vi "Yahoo - Get Data (for stock ticker).vi"(0 "Symbol":string, 3 "error in":errorcluster) -> (6 "Stock Data":T1, 9 "error out":errorcluster)   [LabVIEW 2011]
doc: "Get the symbol data from Yahoo Finance.\n\nInputs:\n Symbol: Stock ticker symbol.\n Error in: Describes error conditions that occur before this node runs. This input provides standard error in functionality.\n\nOutputs:\n Stock Data: Parsed Stock Data\n Symbol\n Name\n Price\n Change\n Change %\n Volume: N/A\n Error out: Contains error information. This output provides standard error out functionality."
uses:
  Stock Data Control.ctl
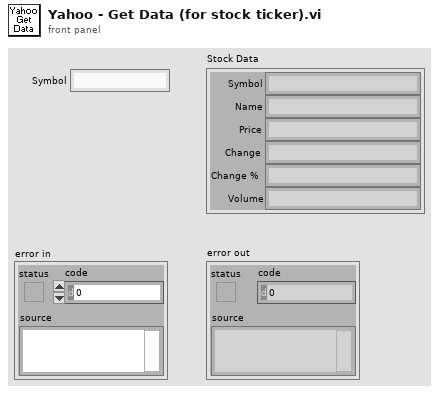
[diagram p1: front panel]
types:
  T1 = typedef "Stock Data Control.ctl" = cluster{"Symbol":string, "Name":string, "Price":string, "Change":string, "Change %":string, "Volume":string}
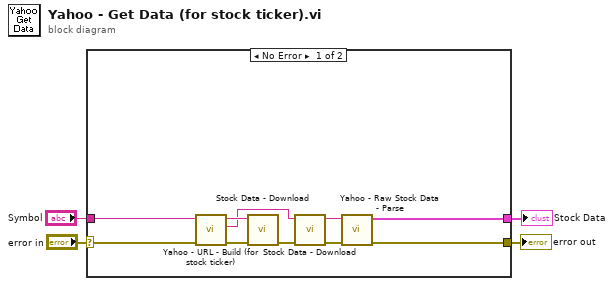
[diagram p0: block diagram]
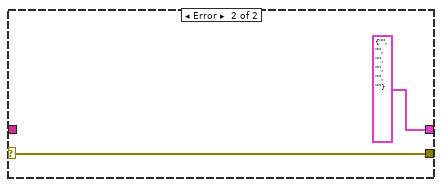
[diagram p2: hidden frame]
diagram:
  n1 = case shown="No Error" "error in" {
    selector: "error in" -> [w8 w16]
    tunnel: [w7 w16] -> w4
    tunnel: [w6 T1 {"Symbol"="", "Name"="", "Price"="", "Change"="", "Change %"="", "Volume"=""} ("Stock Data")] -> w2
    tunnel: "Symbol" -> [w5 _]
    frame No Error {
      n2 = call "Yahoo - URL - Build (for stock ticker).vi"("Symbol"=w5, "error in"=w8) -> ("URL (Pre-redirect)"=w14:string, "URL (Post-redirect)"=w9:string, "error out"=w13:errorcluster)  [unwired: 5 in]
      n3 = call "Stock Data - Download.vi"("error in"=w13, "URL"=w14) -> ("error out"=w12:errorcluster)  [unwired: 7 in, 2 out]
      n4 = call "Stock Data - Download.vi"("error in"=w12, "URL"=w9) -> ("error out"=w11:errorcluster, "Raw Stock Data"=w10:string)  [unwired: 7 in, 1 out]
      n5 = call "Yahoo - Raw Stock Data - Parse.vi"("Raw Stock Data"=w10, "error in"=w11) -> ("Stock Data"=w6:T1, "error out"=w7:errorcluster)  [unwired: 7 in]
    }
    frame Error {
    }
  }
  "error out" <- w4
  "Stock Data" <- w2
